vi "Convert SN bytes to SN data.vi"(11 "SN Data Bytes":u8[](array[numeric]) format="%.0x") -> (3 "SN":u32)   [LabVIEW 2023]
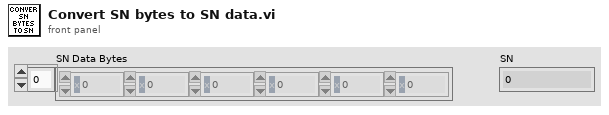
[diagram p1: front panel]
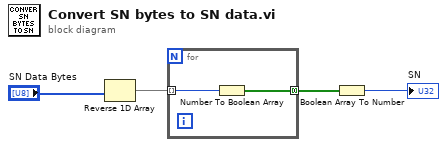
[diagram p0: block diagram]
diagram:
  n1 = Reverse 1D Array(array="SN Data Bytes") -> (reversed array=w3:u8[])
  n2 = for {
    tunnel: w3 -> [w6] mode=indexing
    tunnel: [w5] -> w2 mode=concatenating
    n3 = Number To Boolean Array(number=w6) -> (Boolean array=w5:bool[])
  }
  n4 = Boolean Array To Number(Boolean array=w2) -> (number=→"SN":u32)
